vi "Query.vi"(8 "error in (no error)":errorcluster, 9 "current time":timestamp, 10 "gRPCid":T1) -> (0 "error out":errorcluster)   [LabVIEW 2019, in "ctet_mux_User Library.lvlib"]
uses:
  ctet_mux_User Library.lvlib
  Servers/ctet_mux/gRPC lvSupport/Server API/typeDefs/grpcId.ctl
  Servers/ctet_mux/ctet_mux Class/RPC Messages/measurementservice_QueryResponse/measurementservice_QueryResponse_Data.ctl
  Servers/ctet_mux/ctet_mux Class/ctet_mux.lvclass
  Servers/ctet_mux/gRPC lvSupport/gprc-lvsupport.lvlib
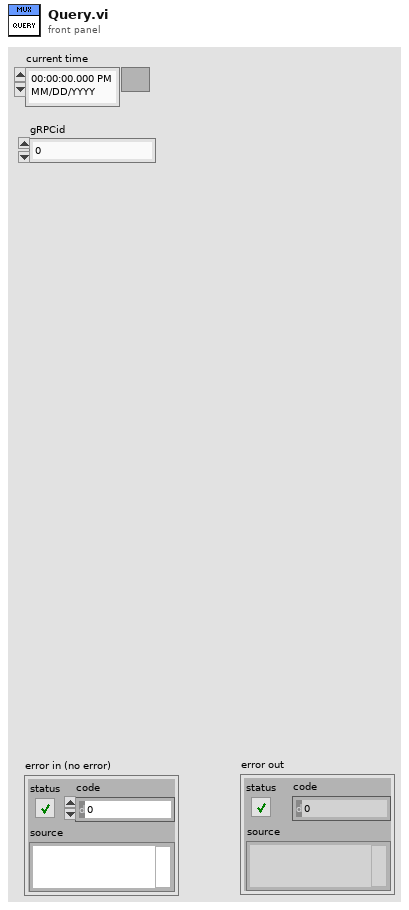
[diagram p1: front panel]
types:
  T1 = typedef "ctet_mux.lvlib/gprc-lvsupport.lvlib/grpcId.ctl" = u64
  T2 = typedef "ctet_mux.lvlib/ctet_mux.lvclass/measurementservice_QueryResponse_Data.ctl" = cluster{"message":string, "status":i64}
  T3 = typedef "ctet_mux.lvlib/ctet_mux.lvclass/measurementservice_QueryRequest_Data.ctl" = cluster{"query":string}
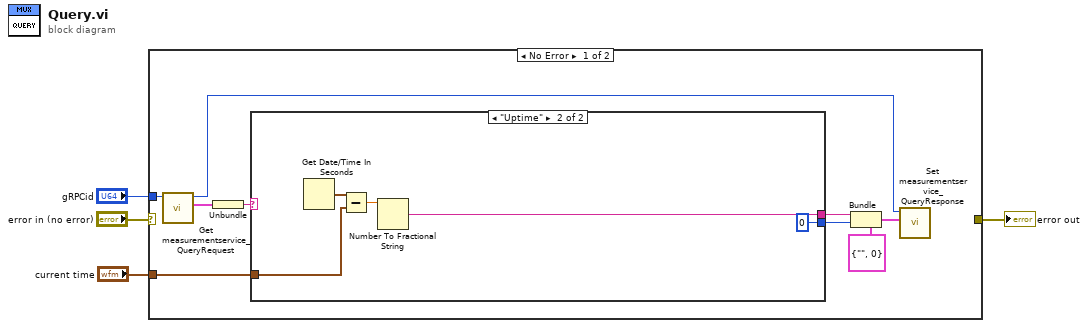
[diagram p0: block diagram]
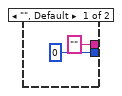
[diagram p2: hidden frame]
diagram:
  n1 = case shown="No Error" "error in (no error)" {
    selector: "error in (no error)" -> [_ w21]
    tunnel: [_ w21] -> w4
    tunnel: "current time" -> [w12 _]
    tunnel: "gRPCid" -> [w9 _]
    frame No Error {
      n2 = call "Get measurementservice_QueryRequest.vi"("gRPCid"=w9) -> ("Message Data"=w8:T3, "gRPCid out"=w5:T1)  [unwired: 8 in, 1 out]
      n3 = Unbundle(w8) -> ("query"=w13:string)
      n4 = case shown="\"Uptime\"" w13 {
        tunnel: w12 -> [_ w19]
        tunnel: ["" w17] -> w11
        tunnel: [i64 0 ("status") i64 0 ("status")] -> w10
        frame "", Default {
        }
        frame "Uptime" {
          n5 = Get Date/Time In Seconds() -> (seconds since 1Jan1904=w20:timestamp)
          n6 = Subtract(x=w20, y=w19) -> (x-y=w18:dbl)
          n7 = Number To Fractional String(number=w18) -> (F-format string=w17:string)  [unwired: 3 in]
        }
      }
      n8 = Bundle(cluster=T2 {"message"="", "status"=0} ("measurementservice_QueryResponse_Data"), "message"=w11, "status"=w10) -> (w6:T2)
      n9 = call "Set measurementservice_QueryResponse.vi"("Message Data"=w6, "gRPCid"=w5) -> ()  [unwired: 9 in, 1 out]
    }
    frame Error {
    }
  }
  "error out" <- w4
